vi "CIGetSetConfig.vi"(7 "Set? (F)":bool, 10 "GenericCameraConfig":T1={"Framerate (Hz)"=60, "Exposure time (us)"=5000, "Image size"={"Width"=1280, "Height"=1024}}, 11 "Camera state":variant) -> (2 "GenericCameraConfig (out)":T1={"Framerate (Hz)"=60, "Exposure time (us)"=5000, "Image size"={"Width"=1280, "Height"=1024}}, 3 "Camera state (out)":variant)   [LabVIEW 2011]
uses:
  BeadTracker2.llb/GenericCameraConfigType.ctl
  mkCameraData.ctl
  CameraConfig.ctl
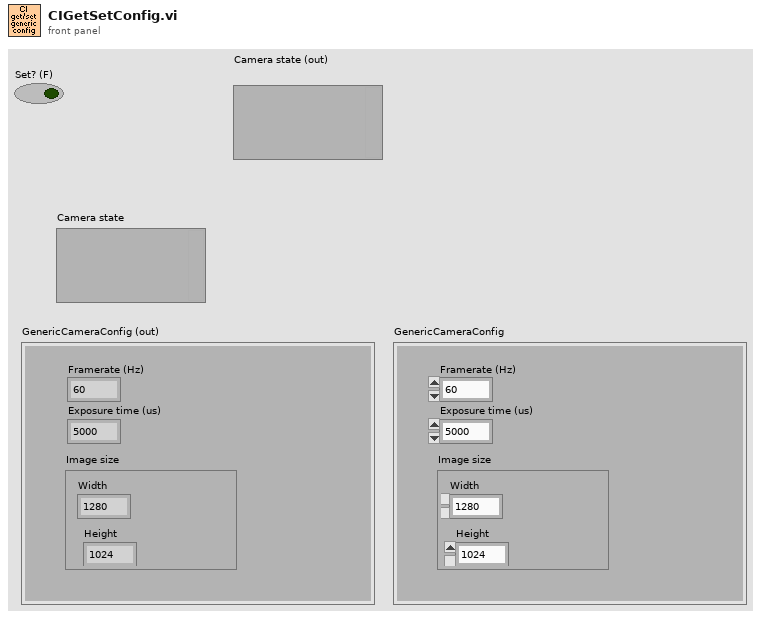
[diagram p1: front panel]
types:
  T1 = typedef "GenericCameraConfigType.ctl" = cluster{"Framerate (Hz)":i32, "Exposure time (us)":i32, "Image size":cluster{"Width":i32, "Height":i32}}
  T2 = typedef "mkCameraData.ctl" = cluster{"Session":refnum<k11>, "Settings":T3}
  T3 = typedef "CameraConfig.ctl" = cluster{"Gain [1-4]":sgl, "Offset":i16, "Mode":i16, "ROIs":cluster{"X":i32, "Y":i32}[], "ROI Size":cluster{"X":i32, "Y":i32}, "Number of buffers":i32, "Use hardware multiple-ROI?":bool, "GenericCameraConfig":T1}
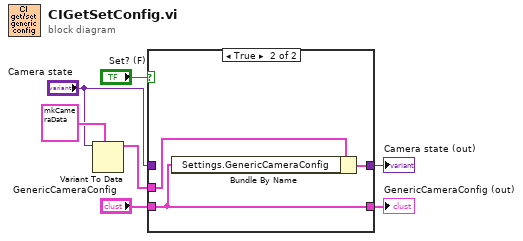
[diagram p0: block diagram]
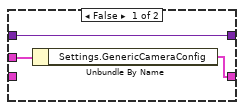
[diagram p2: hidden frame]
diagram:
  n1 = Variant To Data(type=T2 {"Session"=refnum, "Settings"={"Gain [1-4]"=1.0, "Offset"=50, "Mode"=6, "ROIs"=[], "ROI Size"={"X"=0, "Y"=0}, "Number of buffers"=40, "Use hardware multiple-ROI?"=TRUE, "GenericCameraConfig"={"Framerate (Hz)"=60, "Exposure time (us)"=5000, "Image size"={"Width"=1280, "Height"=1024}}}} ("Camera data"), Variant="Camera state") -> (data=w4:T2)  [unwired: 1 in, 1 out]
  n2 = case shown="True" "Set? (F)" {
    tunnel: "GenericCameraConfig" -> [_ w12]
    tunnel: w4 -> [w10 w11]
    tunnel: [w8 w13] -> w3
    tunnel: [w9 w12] -> w2
    tunnel: "Camera state" -> [w8 _]
    frame False {
      n3 = Unbundle By Name(w10) -> ("Settings.GenericCameraConfig"=w9:T1)
    }
    frame True {
      n4 = Bundle By Name(cluster=w11, "Settings.GenericCameraConfig"=w12) -> (w13:T2)
    }
  }
  "GenericCameraConfig (out)" <- w2
  "Camera state (out)" <- w3
